vi "Clear Pending Operation in Remote Control.vi"(8 "error in":errorcluster, 11 "EMS User Interface in":refnum<class "EMS User Interface.lvclass">) -> (0 "error out":errorcluster, 3 "EMS User Interface out":refnum<class "EMS User Interface.lvclass">)   [LabVIEW 2018, in "EMS User Interface Actor.lvlib" / "EMS User Interface.lvclass"]
uses:
  EMS User Interface.lvclass
  EMS User Interface.lvclass/EMS User Interface.ctl
  <vilib>/ActorFramework/Message Enqueuer/Message Enqueuer.lvclass/Message Enqueuer.ctl
  <vilib>/ActorFramework/Message Enqueuer/Enqueue.vi
  Remote Operation/Remote Operation Abstract Messages/Clear Pending Operation Msg/Clear Pending Operation Msg.lvclass
  C:/Program Files (x86)/National Instruments/LabVIEW 2018/vi.lib/ActorFramework/Message/Message.lvclass
  <vilib>/ActorFramework/Message Priority Queue/Priority Enqueue.vi
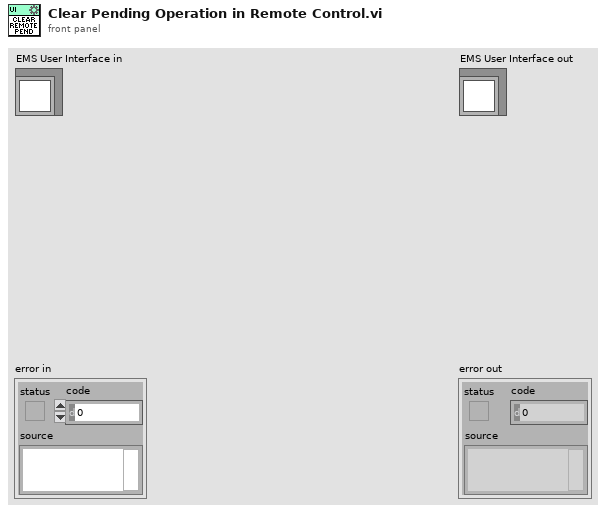
[diagram p1: front panel]
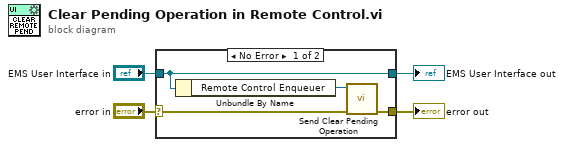
[diagram p0: block diagram]
diagram:
  n1 = case shown="No Error" "error in" {
    selector: "error in" -> [w6 w10]
    tunnel: [w5 w10] -> w3
    tunnel: [w8 w9] -> w1
    tunnel: "EMS User Interface in" -> [w8 w9]
    frame No Error {
      n2 = Unbundle By Name(w8) -> ("Remote Control Enqueuer"=w7:refnum<class "Message Enqueuer.lvclass">)
      n3 = call "Send Clear Pending Operation.vi"("error in (no error)"=w6, "Message Enqueuer"=w7) -> ("error out"=w5:errorcluster)  [unwired: 8 in, 1 out]
    }
    frame Error {
    }
  }
  "error out" <- w3
  "EMS User Interface out" <- w1
